vi "queryFilterStatus.vi"(8 "error in (no error)":errorcluster, 10 "FilterType":enum16{"Average", "Median"}(ring), 11 "Electrometer in":refnum<class "Electrometer.lvclass">) -> (0 "error out":errorcluster, 2 "Filter status":string, 3 "Electrometer out":refnum<class "Electrometer.lvclass">)   [LabVIEW 2016, in "Electrometer.lvclass"]
doc: "Query specific filter status for measuremente mode"
uses:
  Electrometer.lvclass
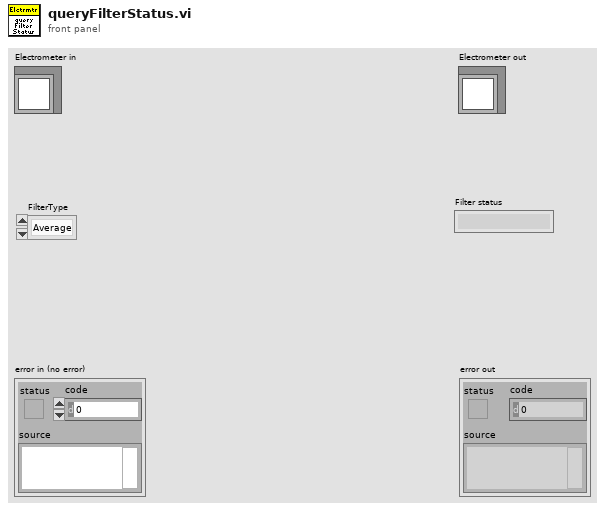
[diagram p1: front panel]
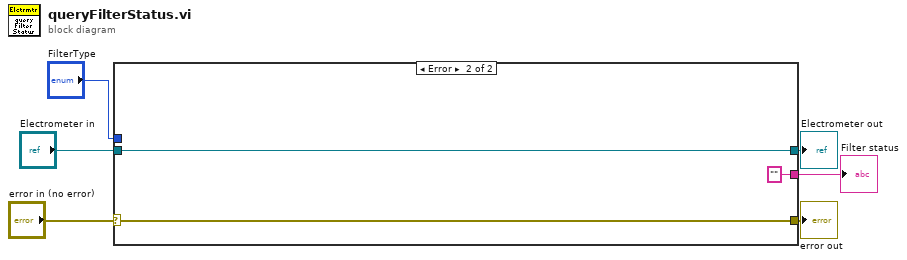
[diagram p0: block diagram]
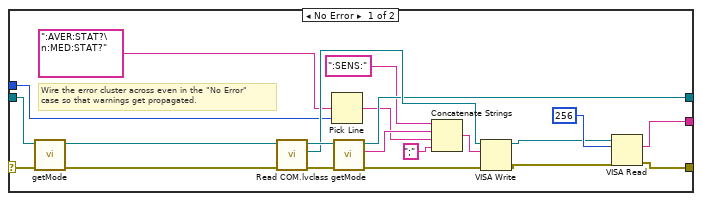
[diagram p2: hidden frame]
diagram:
  n1 = case shown="Error" "error in (no error)" {
    selector: "error in (no error)" -> [w17 w30]
    tunnel: [w8 w30] -> w5
    tunnel: [w19 w29] -> w3
    tunnel: "Electrometer in" -> [w21 w29]
    tunnel: "FilterType" -> [w14 _]
    tunnel: [w7 "" ("read buffer")] -> w1
    frame No Error {
      # "Wire the error cluster across even in the \"No Error\"\ncase so that warnings get propagated."
      n2 = call "getMode.vi"("error in (no error)"=w17, "Electrometer in"=w21) -> ("error out"=w18:errorcluster, "Electrometer out"=w20:refnum<class "Electrometer.lvclass">)  [unwired: 7 in, 1 out]
      n3 = call "Read COM.lvclass.vi"("error in (no error)"=w18, "Electrometer in"=w20) -> ("error out"=w26:errorcluster, "VISA"=w24:refnum<visa-resource-name>, "Electrometer out"=w27:refnum<class "Electrometer.lvclass">)  [unwired: 7 in]
      n4 = Pick Line(multi-line string=":AVER:STAT?\n:MED:STAT?", line index=w14) -> (output string=w12:string)  [unwired: 1 in]
      n5 = call "getMode.vi"("error in (no error)"=w26, "Electrometer in"=w27) -> ("error out"=w23:errorcluster, "Mode"=w25:string, "Electrometer out"=w19:refnum<class "Electrometer.lvclass">)  [unwired: 7 in]
      n6 = Concatenate Strings(":SENS:", w25, w12, ";" ("string")) -> (w22:string)
      n7 = VISA Write(VISA resource name=w24, write buffer=w22, error in (no error)=w23) -> (VISA resource name out=w10:refnum<visa-resource-name>, error out=w9:errorcluster)  [unwired: 1 out]
      n8 = VISA Read(VISA resource name=w10, byte count=u32 256, error in (no error)=w9) -> (read buffer=w7:string, error out=w8:errorcluster)  [unwired: 2 out]
    }
    frame Error {
    }
  }
  "error out" <- w5
  "Electrometer out" <- w3
  "Filter status" <- w1
